vi "PersonnelReportDataToGraph.vi"(8 "error in (no error)":errorcluster, 11 "Array":T1[](array[typedef])=[{"PersonnelName"="d1", "NumRequestsFulfilled"=11, "AvgFulfillTime(s)"=49.18181818181818, "NumReqWithAlarmFulfilled"=3, "NumRequestsAck"=9, "AvgAckTime(s)"=47.333333333333336, "NumReqWithAlarmAck"=2}, {"PersonnelName"="d2", "NumRequestsFulfilled"=1, "AvgFulfillTime(s)"=8.0, "NumReqWithAlarmFulfilled"=0, "NumRequestsAck"=1, "AvgAckTime(s)"=8.0, "NumReqWithAlarmAck"=0}, {"PersonnelName"="n1", "NumRequestsFulfilled"=3, "AvgFulfillTime(s)"=15.0, "NumReqWithAlarmFulfilled"=1, "NumRequestsAck"=2, "AvgAckTime(s)"=15.0, "NumReqWithAlarmAck"=1}, {"PersonnelName"="n2", "NumRequestsFulfilled"=5, "AvgFulfillTime(s)"=9.0, "NumReqWithAlarmFulfilled"=5, "NumRequestsAck"=3, "AvgAckTime(s)"=3.0, "NumReqWithAlarmAck"=0}]) -> (0 "error out":errorcluster, 1 "# Request with Alarm Completed":i32[][](graph), 2 "Average Fullfill Time":dbl[][](graph), 3 "# Request Completed":i32[][](graph), 4 "# Request Ack":i32[][](graph), 5 "# Request with Alarm":i32[][](graph), 6 "Average Ack Time":dbl[][](graph))   [LabVIEW 2015]
uses:
  TypeDef/PersonnelReport.ctl
panel:
  out "Update":bool
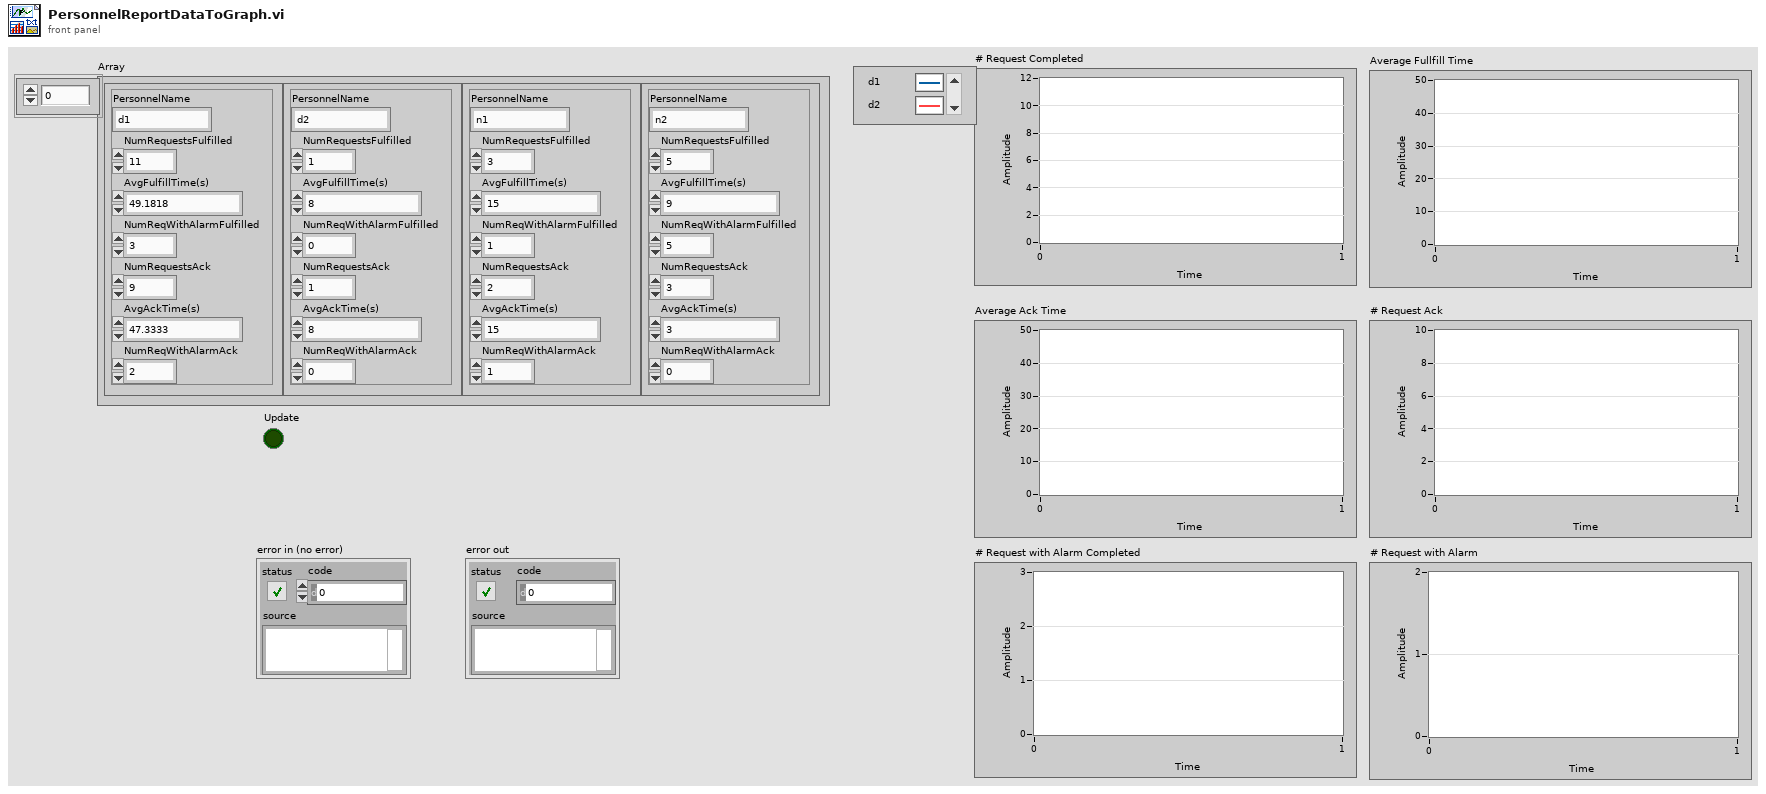
[diagram p1: front panel]
types:
  T1 = typedef "PersonnelReport.ctl" = cluster{"PersonnelName":string, "NumRequestsFulfilled":i32, "AvgFulfillTime(s)":dbl, "NumReqWithAlarmFulfilled":i32, "NumRequestsAck":i32, "AvgAckTime(s)":dbl, "NumReqWithAlarmAck":i32}
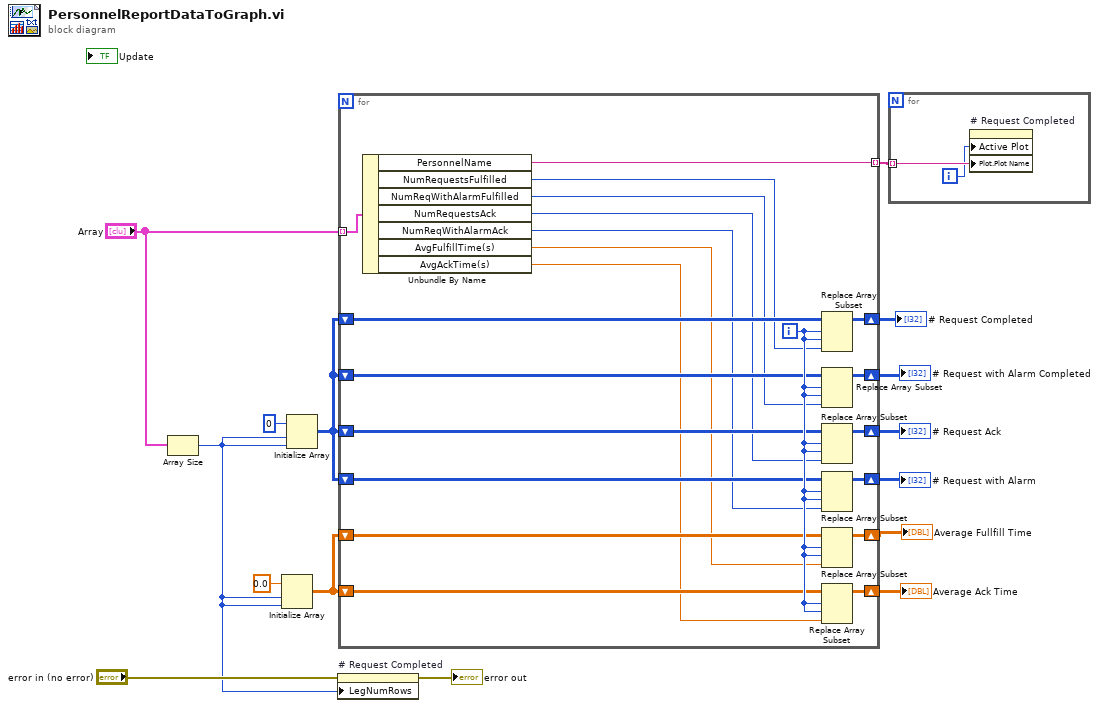
[diagram p0: block diagram]
diagram:
  n1 = Array Size(array="Array") -> (size(s)=w9:i32)
  n2 = Initialize Array(0.0, w9, w9) -> (w7:dbl[][])
  n3 = Initialize Array(0, w9, w9) -> (w8:i32[][])
  n4 = property on="# Request Completed" class="WFGraph (strict)"(error in="error in (no error)", "LegNumRows"=w9) -> (error out=→"error out":errorcluster)  [unwired: 1 in, 1 out]
  n5 = for {
    tunnel: "Array" -> [w36] mode=indexing
    shift-right: [w34] -> w13
    shift-left: w8 -> [w35]
    shift-right: [w31] -> w5
    shift-left: w7 -> [w32]
    shift-right: [w29] -> w2
    shift-left: w8 -> [w30]
    shift-right: [w27] -> w3
    shift-left: w8 -> [w28]
    shift-right: [w23] -> w4
    shift-left: w8 -> [w24]
    shift-right: [w25] -> w6
    shift-left: w7 -> [w26]
    tunnel: [w20] -> w1 mode=indexing
    i -> [w33]
    n6 = Unbundle By Name(w36) -> ("PersonnelName"=w20:string, "NumRequestsFulfilled"=w22:i32, "NumReqWithAlarmFulfilled"=w21:i32, "NumRequestsAck"=w19:i32, "NumReqWithAlarmAck"=w18:i32, "AvgFulfillTime(s)"=w17:dbl, "AvgAckTime(s)"=w16:dbl)
    n7 = Replace Array Subset(array=w35, new element=w22, index (row)=w33, index (col)=w33) -> (w34:i32[][])
    n8 = Replace Array Subset(array=w30, new element=w21, index (row)=w33, index (col)=w33) -> (w29:i32[][])
    n9 = Replace Array Subset(array=w28, new element=w19, index (row)=w33, index (col)=w33) -> (w27:i32[][])
    n10 = Replace Array Subset(array=w24, new element=w18, index (row)=w33, index (col)=w33) -> (w23:i32[][])
    n11 = Replace Array Subset(array=w32, new element=w17, index (row)=w33, index (col)=w33) -> (w31:dbl[][])
    n12 = Replace Array Subset(array=w26, new element=w16, index (row)=w33, index (col)=w33) -> (w25:dbl[][])
  }
  "# Request Completed" <- w13
  "# Request with Alarm Completed" <- w2
  "# Request Ack" <- w3
  "# Request with Alarm" <- w4
  "Average Fullfill Time" <- w5
  "Average Ack Time" <- w6
  n13 = for {
    tunnel: w1 -> [w38] mode=indexing
    i -> [w37]
    n14 = property on="# Request Completed" class="WFGraph (strict)"("Active Plot"=w37, "Plot.Plot Name"=w38) -> ()  [unwired: 2 in, 2 out]
  }
